vi "DAQmx Configure Ref Clock PXIe 100MHz.vi"(0 "DAQmx Task In":refnum<k21>, 11 "error in (no error)":errorcluster) -> (4 "DAQmx Task Out":refnum<k21>, 15 "error out":errorcluster)   [LabVIEW 2020]
doc: "Configures the Reference clock of DAQmx Task to PXIe_CLK100 and rate to 100MHz"
uses:
  <resource>/objmgr/daqmx.rc
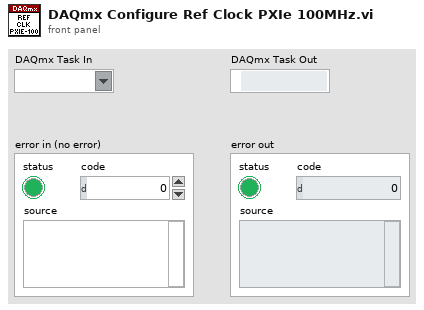
[diagram p1: front panel]
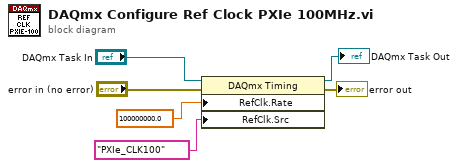
[diagram p0: block diagram]
diagram:
  n1 = property class="DAQmx Timing"(reference="DAQmx Task In", error in="error in (no error)", "RefClk.Rate"=100000000.0, "RefClk.Src"=tag "PXIe_CLK100") -> (reference out=→"DAQmx Task Out":refnum<k21>, error out=→"error out":errorcluster)
